vi "Initialize PJVS.vi"(8 "error in (no error)":errorcluster, 11 "PJVS setup":T1={"PJVS type"=enum."AC-supraVOLTcontrol", "Status Refnum"=refnum, "Abort Refnum"=refnum, "AC-supraVOLTcontrol"={"IP address:port (0.0.0.0:0000)"="0.0.0.0:0000", "Debug mode"=enum."No change", "Timeouts"={"TCP Read & Write (ms)"=7000, "Sensors readout"=5000, "PJVS setup"=10000, "Nullmeter readout"=5000, "Multiplexer setup"=3000, "57XX setup"=15000, "Generator setup"=5000, "Synthesizer setup"=3000, "Sampler readout"=10000}}, "NPL bias source"={"Server name"="CZC", "Bias setup file"=path ""}}) -> (0 "error out":errorcluster, 3 "PJVS setup out":T1={"PJVS type"=enum."AC-supraVOLTcontrol", "Status Refnum"=refnum, "Abort Refnum"=refnum, "AC-supraVOLTcontrol"={"IP address:port (0.0.0.0:0000)"="0.0.0.0:0000", "Debug mode"=enum."No change", "Timeouts"={"TCP Read & Write (ms)"=7000, "Sensors readout"=5000, "PJVS setup"=10000, "Nullmeter readout"=5000, "Multiplexer setup"=3000, "57XX setup"=15000, "Generator setup"=5000, "Synthesizer setup"=3000, "Sampler readout"=10000}}, "NPL bias source"={"Server name"="CZC", "Bias setup file"=path ""}})   [LabVIEW 2020]
doc: "Initialize the PJVS. Calls the initialization routine of the actual driver."
uses:
  Type definitions/PJVS Setup.ctl
  Type definitions/PJVS Type.ctl
  PJVS drivers/acsvcontrol-driver/build/ACSVcontrol-driver_0.2.0.0.llb/Debug status.ctl
  PJVS drivers/acsvcontrol-driver/build/ACSVcontrol-driver_0.2.0.0.llb/Timeouts.ctl
  PJVS drivers/acsvcontrol-driver/build/ACSVcontrol-driver_0.2.0.0.llb/ACSVcontrol-driver.lvlib
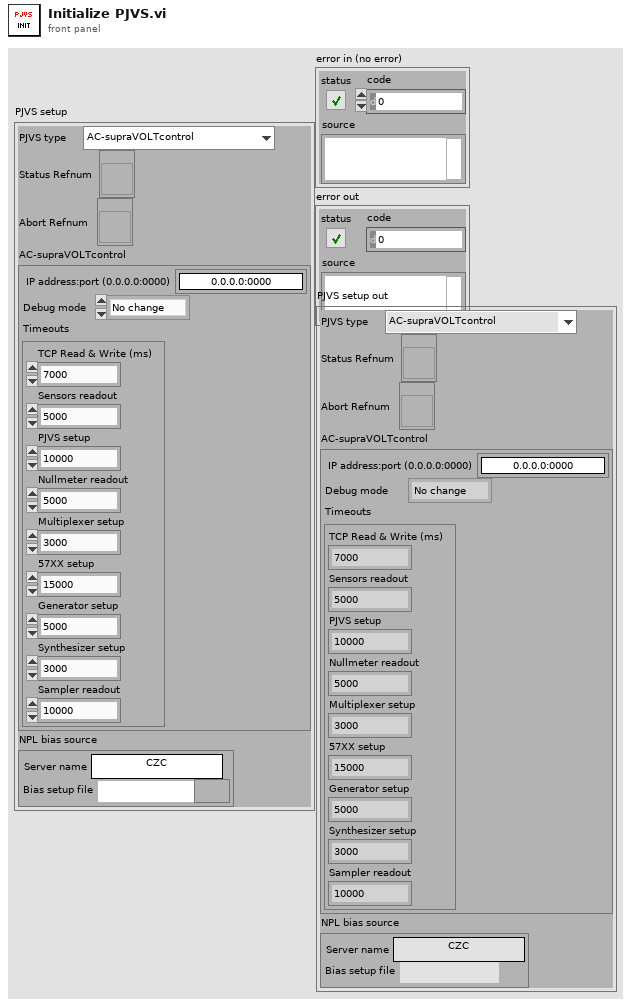
[diagram p1: front panel]
types:
  T1 = typedef "PJVS Setup.ctl" = cluster{"PJVS type":T2, "Status Refnum":refnum<vi>, "Abort Refnum":refnum<vi>, "AC-supraVOLTcontrol":cluster{"IP address:port (0.0.0.0:0000)":string, "Debug mode":T3, "Timeouts":T4}, "NPL bias source":cluster{"Server name":string, "Bias setup file":path}}
  T2 = typedef "PJVS Type.ctl" = enum16{"AC-supraVOLTcontrol", "NPL bias source"}
  T3 = typedef "ACSVcontrol-driver.lvlib/Debug status.ctl" = enum16{"No change", "Off", "On"}
  T4 = typedef "ACSVcontrol-driver.lvlib/Timeouts.ctl" = cluster{"TCP Read & Write (ms)":i32, "Sensors readout":i32, "PJVS setup":i32, "Nullmeter readout":i32, "Multiplexer setup":i32, "57XX setup":i32, "Generator setup":i32, "Synthesizer setup":i32, "Sampler readout":i32}
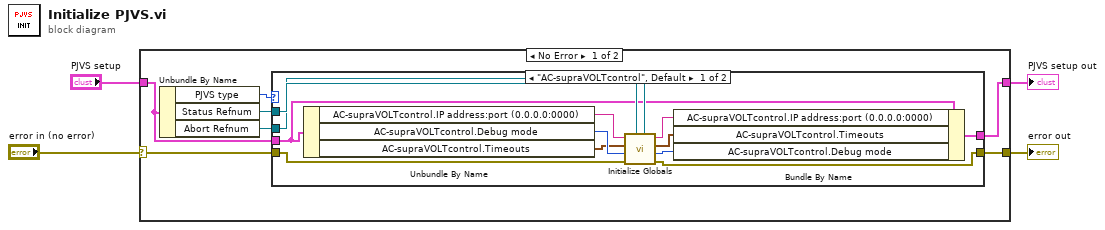
[diagram p0: block diagram]
diagram:
  n1 = case shown="No Error" "error in (no error)" {
    selector: "error in (no error)" -> [w6 w27]
    tunnel: "PJVS setup" -> [w10 w26]
    tunnel: [w7 w27] -> w3
    tunnel: [w5 w26] -> w1
    frame No Error {
      n2 = Unbundle By Name(w10) -> ("PJVS type"=w11:T2, "Status Refnum"=w9:refnum<vi>, "Abort Refnum"=w8:refnum<vi>)
      n3 = case shown="\"AC-supraVOLTcontrol\", Default" w11 {
        tunnel: w10 -> [w16 w24]
        tunnel: w9 -> [w22 _]
        tunnel: w8 -> [w21 _]
        tunnel: w6 -> [w18 w25]
        tunnel: [w17 w25] -> w7
        tunnel: [w12 w24] -> w5
        frame "AC-supraVOLTcontrol", Default {
          n4 = Unbundle By Name(w16) -> ("AC-supraVOLTcontrol.IP address:port (0.0.0.0:0000)"=w23:string, "AC-supraVOLTcontrol.Debug mode"=w20:T3, "AC-supraVOLTcontrol.Timeouts"=w19:T4)
          n5 = call "Initialize Globals.vi"("Abort Refnum"=w21, "Status Refnum"=w22, "error in (pass through)"=w18, "Debug mode"=w20, "Timeouts"=w19, "IP address:port (0.0.0.0:0000)"=w23) -> ("error out"=w17:errorcluster, "Debug mode out"=w13:T3, "Timeouts out"=w14:T4, "IP address:port out"=w15:string)  [unwired: 2 out]
          n6 = Bundle By Name(cluster=w16, "AC-supraVOLTcontrol.IP address:port (0.0.0.0:0000)"=w15, "AC-supraVOLTcontrol.Timeouts"=w14, "AC-supraVOLTcontrol.Debug mode"=w13) -> (w12:T1)
        }
        frame "NPL bias source" {
        }
      }
    }
    frame Error {
    }
  }
  "error out" <- w3
  "PJVS setup out" <- w1
